vi "TSPopup.Close.vi"(8 "error in (no error)":errorcluster) -> (0 "error out":errorcluster)   [LabVIEW 2013]
doc: "Closes the Type Sensitive Popup. Run at end of program.\n\nType Sensitive Popup \nCopyright © 2007, J. David Saunders\nAll rights reserved."
uses:
  Private/TSPopup.Popup Operation.ctl
panel:
  # "Type Sensitive Popup \nCopyright © 2007, J. David Saunders\nAll rights reserved."
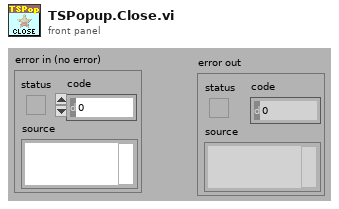
[diagram p1: front panel]
types:
  T1 = typedef "TSPopup.Popup Operation.ctl" = enum16{"Show", "Initialize", "Close", "Popup Done", "Register a Location's Type", "Retrieve Location's Type"}
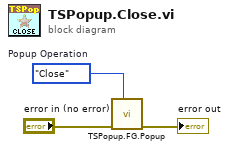
[diagram p0: block diagram]
diagram:
  w3 = TSPopup.Popup_Operation."Close"  # Popup Operation
  n1 = call "TSPopup.FG.Popup.vi"("Popup Operation"=w3, "error in (no error)"="error in (no error)") -> ("error out"=→"error out":errorcluster)  [unwired: 6 in, 3 out]
